vi "Set Path Hex Cfg.vi"(8 "error in (no error)":errorcluster caption="entrée d'erreur (pas d'erreur)", 10 "Path Hex Cfg":path, 11 "Flash_Epox en entrée":refnum<class "Flash_Epox.lvclass">) -> (0 "error out":errorcluster caption="sortie d'erreur", 3 "Flash_Epox en sortie":refnum<class "Flash_Epox.lvclass">)   [LabVIEW 2020, in "Library Test.lvlib" / "Flash_Epox.lvclass"]
uses:
  Flash_Epox.lvclass
  Flash_Epox.lvclass/Flash_Epox.ctl
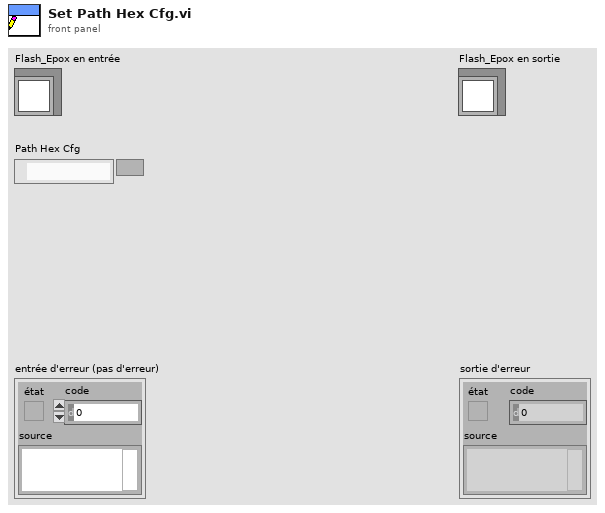
[diagram p1: front panel]
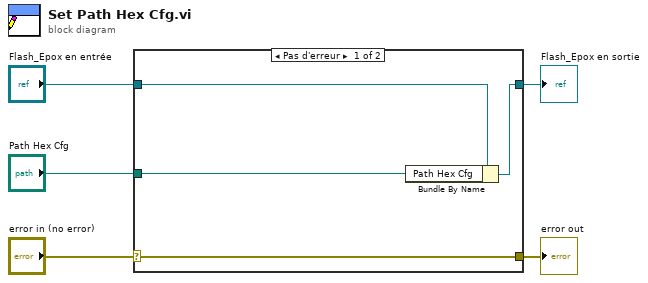
[diagram p0: block diagram]
diagram:
  n1 = case shown="Pas d'erreur" "error in (no error)" {
    selector: "error in (no error)" -> [w9 w10]
    tunnel: [w9 w10] -> w4
    tunnel: [w7 w11] -> w2
    tunnel: "Flash_Epox en entrée" -> [w8 w11]
    tunnel: "Path Hex Cfg" -> [w6 _]
    frame No Error {
      n2 = Bundle By Name(cluster=w8, "Path Hex Cfg"=w6) -> (w7:refnum<class "Flash_Epox.lvclass">)
    }
    frame Error {
    }
  }
  "error out" <- w4
  "Flash_Epox en sortie" <- w2
